vi "Hardware In - NI 9411-2 (Digital Input).vi"(11 "FPGA Ref":T1) -> (3 "NI9411-2":T2)   [LabVIEW 2015, in "ECS-RT.lvlib"]
uses:
  ECS-RT.lvlib
  Typedefs/Raw Inputs/NI9411.ctl
  Typedefs/Raw Inputs/PPWData.ctl
  Typedefs/FPGA Refs/Generic FPGA Ref.ctl
  <vilib>/Utility/error.llb/Error Cluster From Error Code.vi
  <vilib>/rvi/errors/niLvFpgaAdjustHostInterfaceError.vi
  <vilib>/rvi/interface/nirviReadWriteControl/nirviReadWriteControl.xnode
  <vilib>/rvi/interface/Simulation/niFpgaSimulationCallBeginRW.vi
  ECS-Shared.lvlib
  NiFpgaLv.dll
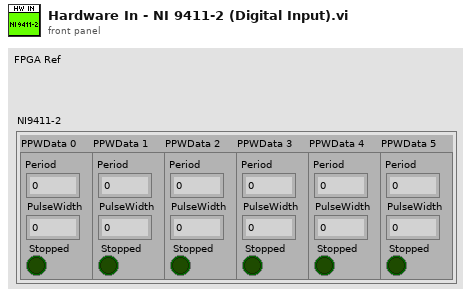
[diagram p1: front panel]
types:
  T1 = typedef "ECS-Shared.lvlib/Generic FPGA Ref.ctl" = refnum<k20>
  T2 = typedef "ECS-Shared.lvlib/NI9411.ctl" = cluster{"PPWData 0":T3, "PPWData 1":T3, "PPWData 2":T3, "PPWData 3":T3, "PPWData 4":T3, "PPWData 5":T3}
  T3 = typedef "ECS-Shared.lvlib/PPWData.ctl" = cluster{"Period":u32, "PulseWidth":u32, "Stopped":bool}
  T4 = cluster{"Period":u32, "PulseWidth":u32, "Stopped":bool}
  T5 = cluster{"Period":u32, "PulseWidth":u32, "Stopped":bool}[]
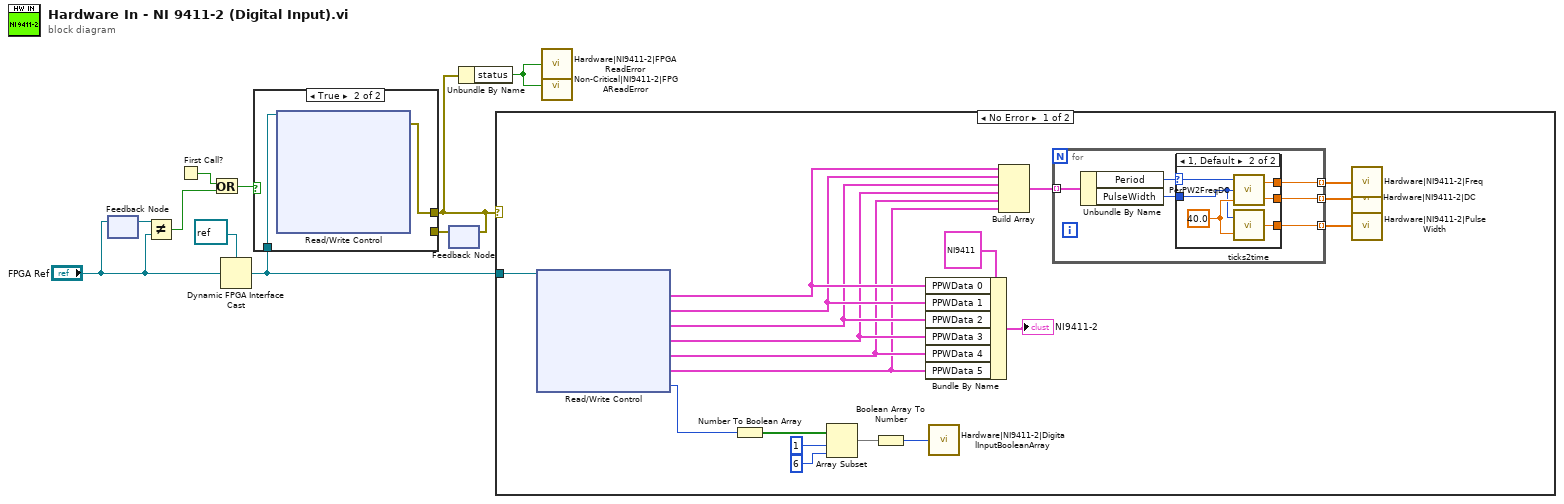
[diagram p0: block diagram]
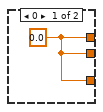
[diagram p3: hidden frame]
diagram:
  n1 = feedback #1() -> (w9:T1)  [unwired: 1 in]
  n2 = feedback-in #1("FPGA Ref") -> ()
  n3 = Not Equal?(x=w9, y="FPGA Ref") -> (x != y?=w10:bool)
  n4 = First Call?() -> (First Call?: T/F=w8:bool)
  n5 = Or(x=w8, y=w10) -> (x .or. y?=w7:bool)
  n6 = Dynamic FPGA Interface Cast(Session In=refnum<k20> refnum ("FPGA VI Reference Out"), Type="FPGA Ref") -> (Session Out=w3:refnum<k20>)
  n7 = feedback #2() -> (w6:errorcluster)  [unwired: 1 in]
  n8 = case shown="True" w7 {
    tunnel: [w11 w12] -> w2
    tunnel: w6 -> [w11 _]
    tunnel: w3 -> [_ w13]
    frame False {
    }
    frame True {
      n9 = xnode "Read/Write Control"("FPGA VI Reference In"=w13) -> ("error out"=w12:errorcluster)  [unwired: 1 in, 8 out]
    }
  }
  n10 = feedback-in #2(w2) -> ()
  n11 = Unbundle By Name(w2) -> ("status"=w1:bool)
  n12 = case shown="No Error" w2 {
    tunnel: w3 -> [w21 _]
    frame No Error {
      n13 = xnode "Read/Write Control"("FPGA VI Reference In"=w21) -> ("9411-2.0.PPWData"=w20:T4, "9411-2.1.PPWData"=w19:T4, "9411-2.2.PPWData"=w18:T4, "9411-2.3.PPWData"=w17:T4, "9411-2.4.PPWData"=w16:T4, "9411-2.5.PPWData"=w15:T4, "9411-2.DigitalTriggers"=w14:u32)  [unwired: 1 in, 2 out]
      n14 = Number To Boolean Array(number=w14) -> (Boolean array=w22:bool[])
      n15 = Array Subset(array=w22, index=1, length=6) -> (w25:bool[])
      n16 = Boolean Array To Number(Boolean array=w25) -> (number=w26:u32)
      n17 = Bundle By Name(cluster=T2 {"PPWData 0"={"Period"=0, "PulseWidth"=0, "Stopped"=FALSE}, "PPWData 1"={"Period"=0, "PulseWidth"=0, "Stopped"=FALSE}, "PPWData 2"={"Period"=0, "PulseWidth"=0, "Stopped"=FALSE}, "PPWData 3"={"Period"=0, "PulseWidth"=0, "Stopped"=FALSE}, "PPWData 4"={"Period"=0, "PulseWidth"=0, "Stopped"=FALSE}, "PPWData 5"={"Period"=0, "PulseWidth"=0, "Stopped"=FALSE}} ("9411-1"), "PPWData 0"=w20, "PPWData 1"=w19, "PPWData 2"=w18, "PPWData 3"=w17, "PPWData 4"=w16, "PPWData 5"=w15) -> (→"NI9411-2":T2)
      n18 = call "Hardware|NI9411-2|DigitalInputBooleanArray"("Value"=w26) -> ()
      n19 = Build Array(w20, w19, w18, w17, w16, w15) -> (w32:T5)
      n20 = for {
        tunnel: w32 -> [w37] mode=indexing
        tunnel: [w34] -> w31 mode=indexing
        tunnel: [w35] -> w30 mode=indexing
        tunnel: [w36] -> w29 mode=indexing
        n21 = Unbundle By Name(w37) -> ("Period"=w33:u32, "PulseWidth"=w38:u32)
        n22 = case shown="1, Default" w33 {
          selector: w33 -> [_ w40]
          tunnel: w38 -> [_ w44]
          tunnel: [w39 w43] -> w36
          tunnel: [w39 w42] -> w35
          tunnel: [w39 w41] -> w34
          frame 0 {
            w39 = sgl 0.0 ("Frequency(Hz)")
          }
          frame 1, Default {
            w45 = sgl 40.0 ("Clock Frequency (MHz, 40)")
            n23 = call <vilib>:"PerPW2FreqDC.vi"("Clock Frequency (MHz, 40)"=w45, "PulseWidth(ticks)"=w44, "Period(ticks)"=w40) -> ("DutyCycle(%)"=w42:sgl, "Frequency(Hz)"=w41:sgl)
            n24 = call <vilib>:"ticks2time.vi"("Clock Frequency (MHz, 40)"=w45, "Ticks"=w44) -> ("Time (msec)"=w43:sgl)
          }
        }
      }
      n25 = call "Hardware|NI9411-2|Freq"("Value"=w31) -> ()
      n26 = call "Hardware|NI9411-2|DC"("Value"=w30) -> ()
      n27 = call "Hardware|NI9411-2|PulseWidth"("Value"=w29) -> ()
    }
    frame Error {
    }
  }
  n28 = call "Hardware|NI9411-2|FPGAReadError"("Value"=w1) -> ()
  n29 = call "Non-Critical|NI9411-2|FPGAReadError"("Fault"=w1) -> ()  [unwired: 2 in]
